vi "Write to the MONO.vi"(4 "MONOCHOMATOR":refnum<visa-resource-name>, 10 "write buffer":string) -> (0 "error out":errorcluster, 6 "read buffer":string, 7 "VISA resource name out":refnum<visa-resource-name>)   [LabVIEW 2024]
panel:
  in  "error in":errorcluster
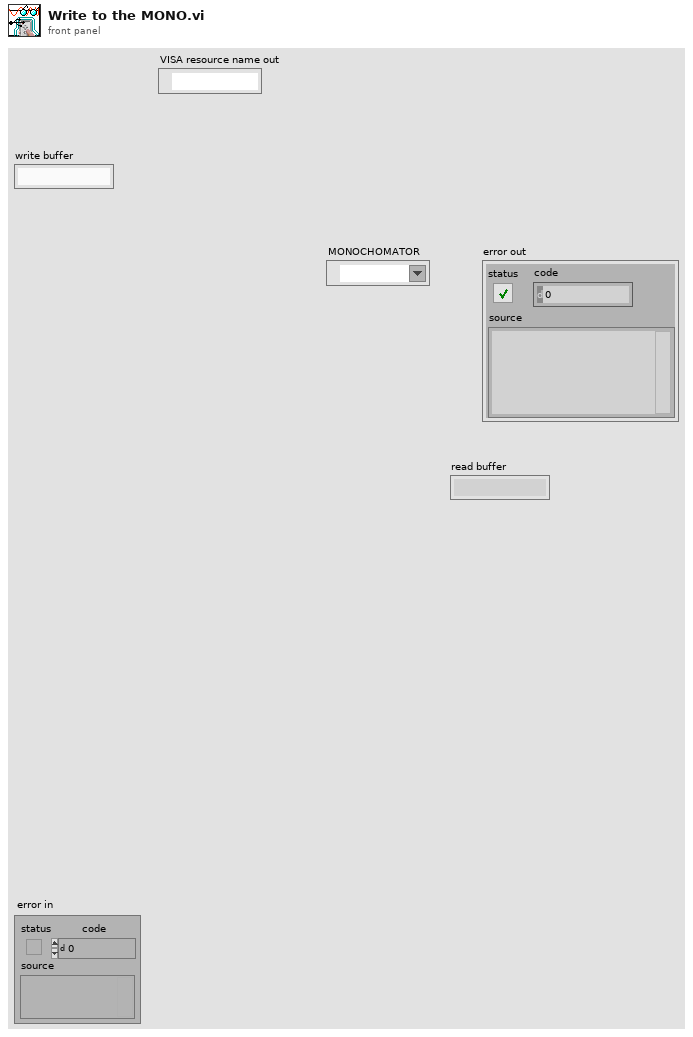
[diagram p1: front panel]
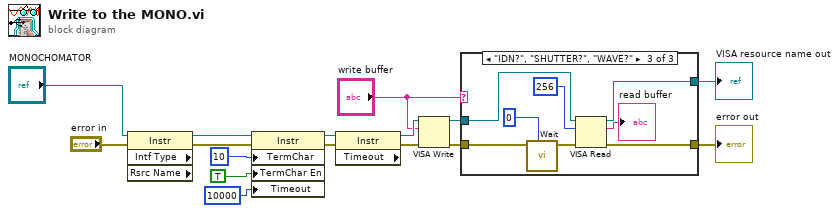
[diagram p0: block diagram]
diagram:
  n1 = property class="Instr" props=["Intf Type", "Rsrc Name"](reference="MONOCHOMATOR", error in="error in") -> (reference out=w16:refnum<visa-resource-name>, error out=w14:errorcluster)  [unwired: 2 out]
  n2 = property class="Instr"(reference=w16, error in=w14, "TermChar"=u8 10 ("Message Based Settings:Termination Character"), "TermChar En"=TRUE ("Message Based Settings:Termination Character Enable"), "Timeout"=u32 10000 ("General Settings:Timeout Value")) -> (reference out=w6:refnum<visa-resource-name>, error out=w5:errorcluster)
  n3 = property class="Instr" props=["Timeout"](reference=w6, error in=w5) -> (reference out=w12:refnum<visa-resource-name>, error out=w11:errorcluster)  [unwired: 1 out]
  n4 = VISA Write(VISA resource name=w12, write buffer="write buffer", error in (no error)=w11) -> (VISA resource name out=w4:refnum<visa-resource-name>, error out=w10:errorcluster)  [unwired: 1 out]
  n5 = case shown="\"IDN?\", \"SHUTTER?\", \"WAVE?\"" "write buffer" {
    tunnel: w10 -> [w17 w19 w28]
    tunnel: w4 -> [w18 w20 w26]
    tunnel: [w17 w19 w24] -> w3
    tunnel: [w18 w20 w23] -> w2
    frame "False", Default {
    }
    frame "GOWAVE", "SHUTTER C", "SHUTTER O" {
    }
    frame "IDN?", "SHUTTER?", "WAVE?" {
      n6 = call "Wait.vi"("milliseconds to wait"=u32 0, "Error In"=w28) -> ("Error Out"=w25:errorcluster)  [unwired: 9 in]
      n7 = VISA Read(VISA resource name=w26, byte count=u32 256, error in (no error)=w25) -> (VISA resource name out=w23:refnum<visa-resource-name>, read buffer=→"read buffer":string, error out=w24:errorcluster)  [unwired: 1 out]
    }
  }
  "error out" <- w3
  "VISA resource name out" <- w2
